vi "Scripting.vi"   [LabVIEW 2020]
uses:
  <vilib>/Utility/traverseref.llb/TRef TravTarget.ctl
  <vilib>/event_ctls.llb/lveventtype.ctl
types:
  T1 = typedef "TRef TravTarget.ctl" = enum16{"FP", "BD", "Other"}
  T2 = typedef "lveventtype.ctl" = enum32{"Null", "Timeout", "Annotation Menu Selection", "Annotation Menu Selection?", "App Instance Close", "App Instance Close?", "Autoscale Range Change", "Bookmark Info Change", "Cell Edit", "Cell Edit?", "Cursor Grab", "Cursor Grab?", "Cursor Menu Selection", "Cursor Menu Selection?", "Cursor Move", "Cursor Release", "Data Change", "Direction Change", "Display State Change", "Drag Ended", "Drag Enter", "Drag Leave", "Drag Over", "Drag Source Update", "Drag Starting", "Drag Starting?", "Drop", "Exec State Change", "Key Down", "Key Down?", "Key Repeat", "Key Repeat?", "Key Up", "Listbox Double Click", "Menu Activation?", "Menu Selection (App)", "Menu Selection? (App)", "Menu Selection (User)", "Mouse Down", "Mouse Down?", "Mouse Enter", "Mouse Leave", "Mouse Move", "Mouse Up", "Mouse Wheel", "NI Security User Change (App)", "Pane Size", "Panel Close", "Panel Close?", "Panel Resize", "Plot Attribute Change", "Scale Range Change", "Shortcut Menu Activation?", "Shortcut Menu Selection (App)", "Shortcut Menu Selection? (App)", "Shortcut Menu Selection (User)", "Tree Double Click", "Tree Drag", "Tree Drag?", "Tree Drop", "Tree Drop?", "Tree Item Close", "Tree Item Close?", "Tree Item Open", "Tree Item Open?", "User Event", "Value Change"}
  T3 = cluster{"Event Type":T2, "Limit (-1=none)":i32, "Lock Panel?":bool}
  T4 = cluster{"Event Type":T2, "Limit (-1=none)":i32, "Lock Panel?":bool}[]
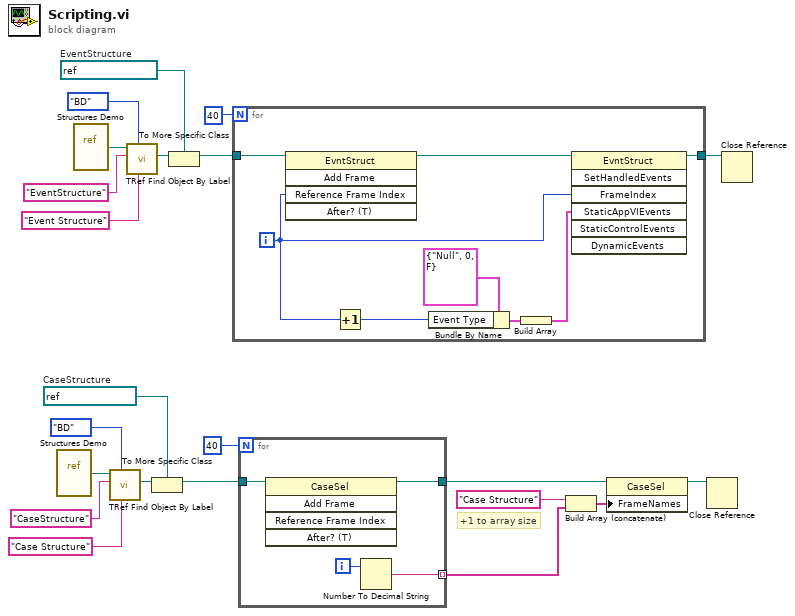
[diagram p0: block diagram]
diagram:
  w8 = refnum<vi> refnum  # CaseStructure
  w18 = refnum<vi> refnum  # EventStructure
  # "+1 to array size"
  n1 = vi-ref "Structures Demo.vi"() -> (w9:refnum<vi>)
  n2 = vi-ref "Structures Demo.vi"() -> (w22:refnum<vi>)
  n3 = call <vilib>:"TRef Find Object By Label.vi"("Label"="Case Structure", "Traverse Target"=TRef_TravTarget."BD", "Class Name"="CaseStructure", "VI Ref"=w9) -> ("Found Obj Ref"=w12:refnum<vi>)  [unwired: 4 in, 3 out]
  n4 = call <vilib>:"TRef Find Object By Label.vi"("Label"="Event Structure", "Traverse Target"=TRef_TravTarget."BD", "Class Name"="EventStructure", "VI Ref"=w22) -> ("Found Obj Ref"=w19:refnum<vi>)  [unwired: 4 in, 3 out]
  n5 = To More Specific Class(target class=w8, reference=w12) -> (specific class reference=w7:refnum<vi>)  [unwired: 1 in, 1 out]
  n6 = To More Specific Class(target class=w18, reference=w19) -> (specific class reference=w15:refnum<vi>)  [unwired: 1 in, 1 out]
  n7 = for {
    N: 40 -> [_]
    tunnel: w15 -> [w24]
    tunnel: [w23] -> w14
    i -> [w25]
    n8 = invoke class="EvntStruct" method="Add Frame"(reference=w24, "Reference Frame Index"=w25) -> (reference out=w30:refnum<vi>)  [unwired: 3 in, 4 out]
    n9 = Increment(x=w25) -> (x+1=w28:i32)
    n10 = Bundle By Name(cluster=T3 {"Event Type"=enum."Null", "Limit (-1=none)"=0, "Lock Panel?"=FALSE} ("Static App/VI Events"), "Event Type"=w28) -> (w27:T3)
    n11 = Build Array(w27) -> (w26:T4)
    n12 = invoke class="EvntStruct" method="SetHandledEvents"(reference=w30, "FrameIndex"=w25, "StaticAppVIEvents"=w26) -> (reference out=w23:refnum<vi>)  [unwired: 4 in, 6 out]
  }
  n13 = for {
    N: 40 -> [_]
    tunnel: w7 -> [w34]
    tunnel: [w31] -> w6
    tunnel: [w32] -> w4 mode=indexing
    i -> [w33]
    n14 = invoke class="CaseSel" method="Add Frame"(reference=w34) -> (reference out=w31:refnum<vi>)  [unwired: 4 in, 4 out]
    n15 = Number To Decimal String(number=w33) -> (decimal integer string=w32:string)  [unwired: 1 in]
  }
  n16 = Build Array (concatenate)("Case Structure" ("Label"), w4) -> (w2:string[])
  n17 = property class="CaseSel"(reference=w6, "FrameNames"=w2) -> (reference out=w1:refnum<vi>)  [unwired: 1 in, 1 out]
  n18 = Close Reference(reference=w1) -> ()  [unwired: 1 in, 1 out]
  n19 = Close Reference(reference=w14) -> ()  [unwired: 1 in, 1 out]
